vi "Main.vi"(11 "Module Admin":refnum<class "Delacor_lib_QMH_Module Admin.lvclass">) -> ()   [LabVIEW 2018, in "MainInterface.lvlib"]
doc: "This template is based off of the Queued Message Handler design pattern and the Queued Message Handler project template that ships with LabVIEW.\n\nThe main difference is that the queue is private to this module and communication between modules is performed via Broadcast and Request events.\n\nRequest events are wrapped in public API methods and are handled in the Event Handling Loop (EHL) of this VI. Any module can register for Broadcast events sent by this module. The EHL generates messages based on user interface actions.\n\nThe Message Handling Loop (MHL) processes messages generated by the EHL, or by other messages. The messages are string values, so new messages can be added easily to the Message Cases case structure in the MHL. Each message cluster can also provide an optional value for Message Data, which is a variant that can be converted to whatever message-specific data is required.\n_____\nBased on DQMH Project Template 7.0.1.1316."
uses:
  MainInterface.lvlib
  <vilib>/Delacor/Delacor QMH/Libraries/Module Admin_class/Delacor_lib_QMH_Module Admin.lvclass
  User Interface/Status Light Bar.ctl
  User Interface/User Interface.lvclass
  <vilib>/Delacor/Delacor QMH/Libraries/Message Queue_class/Delacor_lib_QMH_Message Queue.lvclass/Delacor_lib_QMH_Message Queue.ctl
  Launch Function Argument.ctl
  Stop Argument--cluster.ctl
  Register Window Argument--cluster.ctl
  <vilib>/Delacor/Delacor QMH/Libraries/Message Queue_class/Delacor_lib_QMH_Message Queue.lvclass
  Unregister Window Argument--cluster.ctl
  Is Window Opened Argument--cluster.ctl
  Is Window Opened (Reply Payload)--cluster.ctl
  Disbale Item Argument--cluster.ctl
  Enable Item Argument--cluster.ctl
  <vilib>/Utility/miscctls.llb/LVPointTypeDef.ctl
  <vilib>/Delacor/Delacor QMH/Libraries/Module Admin_class/Delacor_lib_QMH_Module Admin.lvclass/Delacor_lib_QMH_Module Admin.ctl
  <vilib>/Delacor/Delacor QMH/Libraries/Message Queue_class/Delacor_lib_QMH_Enqueue Message (Single).vi
  <vilib>/Delacor/Delacor QMH/Libraries/Module Admin_class/Delacor_lib_QMH_Get External Launch.vi
  ModuleInterface/ModuleInterface.lvlib
panel:
  in  "Status Light Bar":T1=enum."Green"
  in  "min":bool
  in  "close":bool
  out "error out":errorcluster
  out "Status":string
  in  "Simulate MHL Error":bool
  in  "Simulate EHL Error":bool
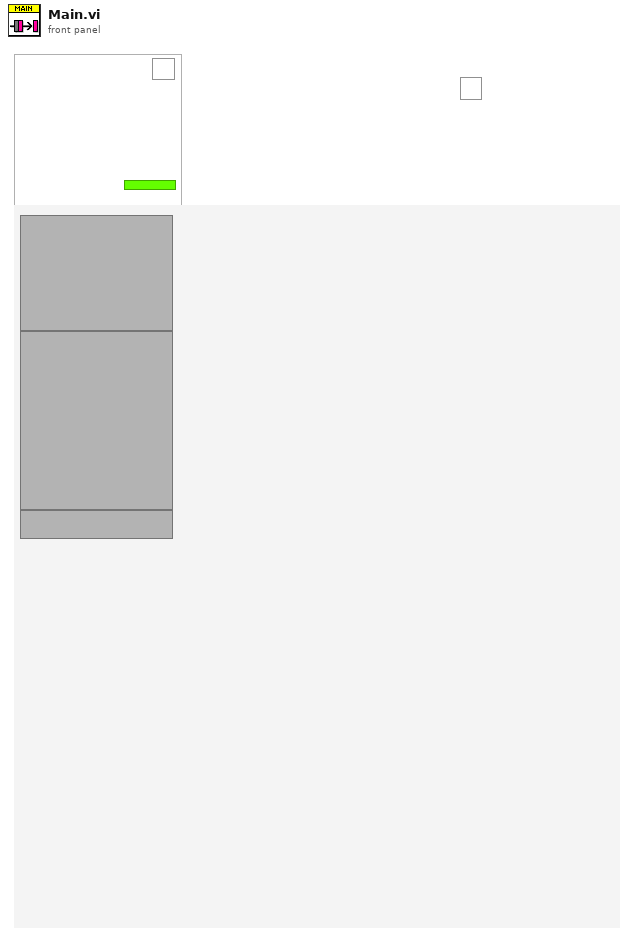
[diagram p1: front panel]
types:
  T1 = typedef "MainInterface.lvlib/User Interface.lvclass/Status Light Bar.ctl" = enum32{"Red", "Yellow", "Green"}
  T2 = typedef "MainInterface.lvlib/Request Events--cluster.ctl" = cluster{"Stop Module":refnum<user-event>, "Show Panel":refnum<user-event>, "Hide Panel":refnum<user-event>, "Get Module Execution Status":refnum<user-event>, "Show Diagram":refnum<user-event>, "Register Window":refnum<user-event>, "Unregister Window":refnum<user-event>, "Is Window Opened":refnum<user-event>, "Disbale Item":refnum<user-event>, "Enable Item":refnum<user-event>}
  T3 = typedef "ModuleInterface.lvlib/ModuleDefinition.ctl" = cluster{"模块名称":string, "项定义":T4[]}
  T4 = typedef "ModuleInterface.lvlib/FunctionItem.ctl" = cluster{"项名":string, "符号图形路径":path}
  T5 = typedef "ModuleInterface.lvlib/Broadcast Events--cluster.ctl" = cluster{"Module Did Init":refnum<user-event>, "Status Updated":refnum<user-event>, "Error Reported":refnum<user-event>, "Module Did Stop":refnum<user-event>, "Update Module Execution Status":refnum<user-event>, "Function Selected":refnum<user-event>, "Window Size Changed":refnum<user-event>}
  T6 = typedef "MainInterface.lvlib/Launch Function Argument.ctl" = cluster{"Module ID":i32, "Module Name":string, "Item Name":string}
  T7 = enum32{"invalid lock state", "Not Locked", "Locked (No Password)", "Password-protected"}
  T8 = typedef "MainInterface.lvlib/Stop Argument--cluster.ctl" = cluster{"Origin":string, "Exit via Stop Module Req?":bool, "Wait for Module to stop?":bool}
  T9 = typedef "MainInterface.lvlib/Register Window Argument--cluster.ctl" = cluster{"Name":string, "Reference":refnum<vi>, "Message Queue":refnum<class "Delacor_lib_QMH_Message Queue.lvclass">}
  T10 = typedef "MainInterface.lvlib/Unregister Window Argument--cluster.ctl" = cluster{"Window Name":string}
  T11 = typedef "MainInterface.lvlib/Is Window Opened Argument--cluster.ctl" = cluster{"Window Name":string, "Wait Notifier":refnum<notifier>, "wait for reply":bool}
  T12 = typedef "MainInterface.lvlib/Disbale Item Argument--cluster.ctl" = cluster{"Module Name":string, "Item Name":string}
  T13 = typedef "MainInterface.lvlib/Enable Item Argument--cluster.ctl" = cluster{"Module Name":string, "Item Name":string}
  T14 = enum32{"Invalid", "Standard", "Closed", "Hidden", "Minimized", "Maximized"}
  T15 = typedef "MainInterface.lvlib/Is Window Opened (Reply Payload)--cluster.ctl" = cluster{"Opened？":bool, "error":errorcluster}
  T16 = typedef "LVPointTypeDef.ctl" = cluster{"Horizontal":i16, "Vertical":i16}
  T17 = typedef "LVRectTypeDef.ctl" = cluster{"Left":i16, "Top":i16, "Right":i16, "Bottom":i16}
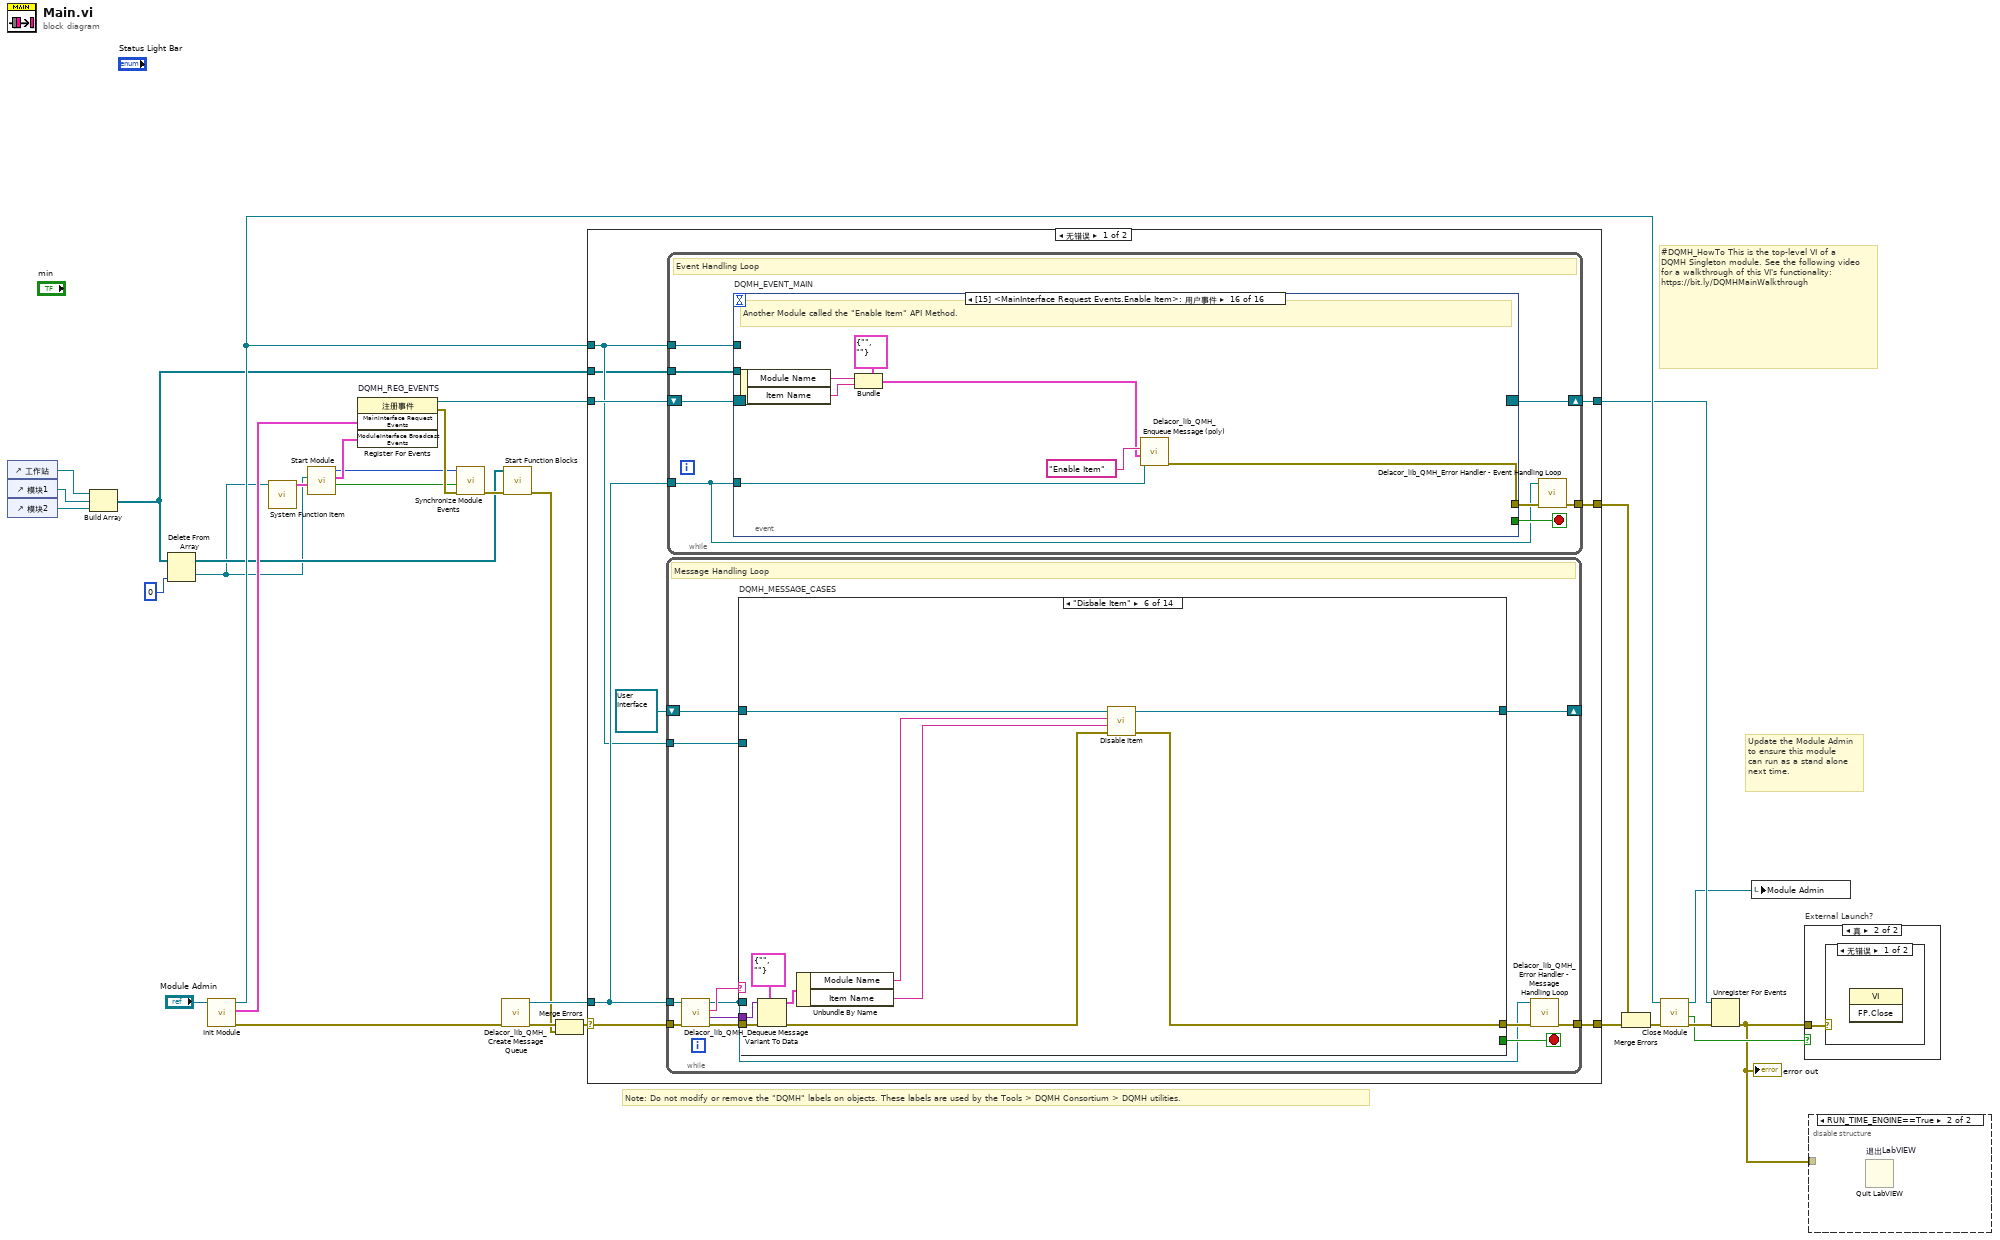
[diagram p0: block diagram]
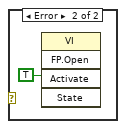
[diagram p4: hidden frame]
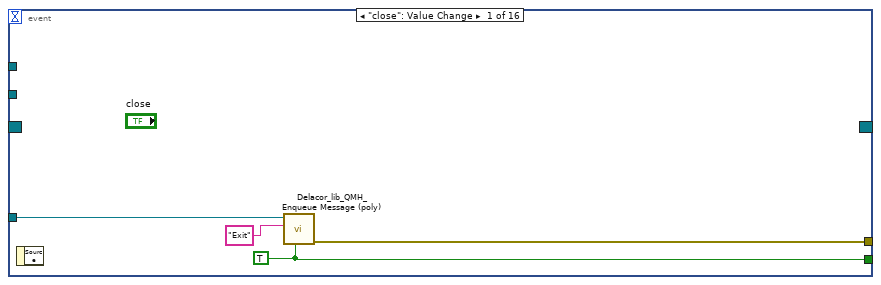
[diagram p5: hidden frame]
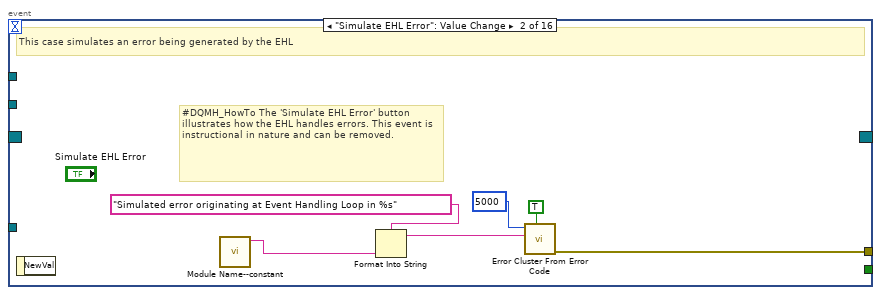
[diagram p6: hidden frame]
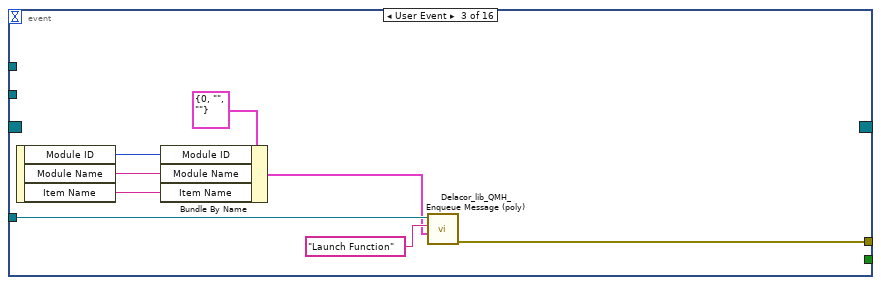
[diagram p7: hidden frame]
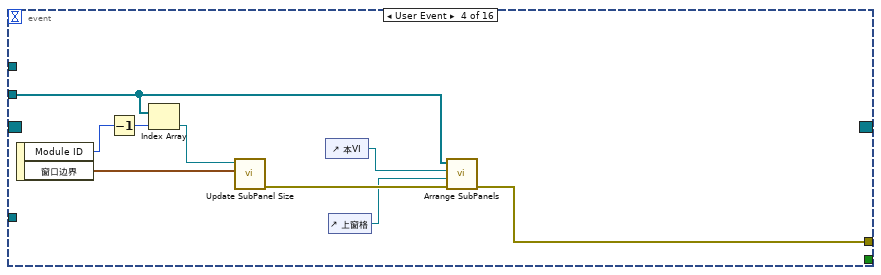
[diagram p8: hidden frame]
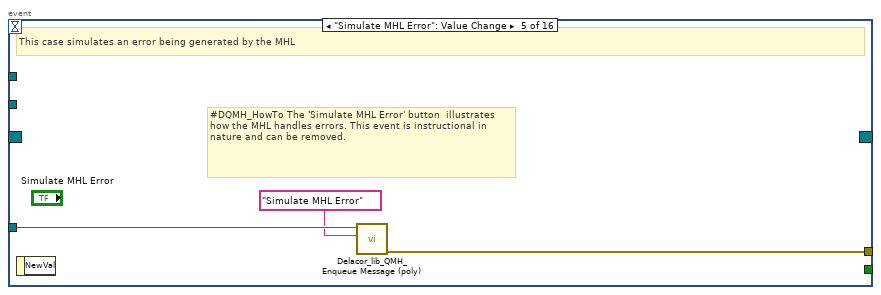
[diagram p9: hidden frame]
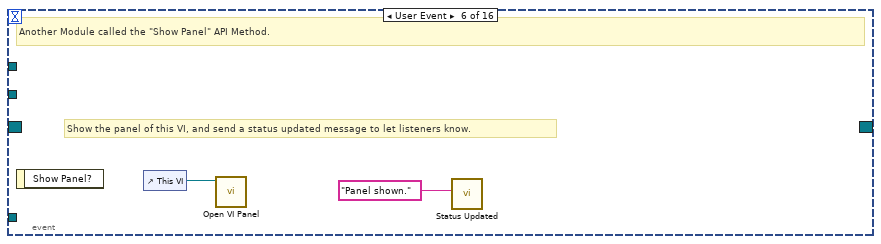
[diagram p10: hidden frame]
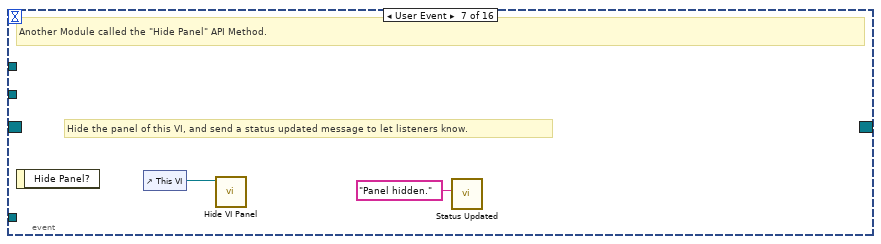
[diagram p11: hidden frame]
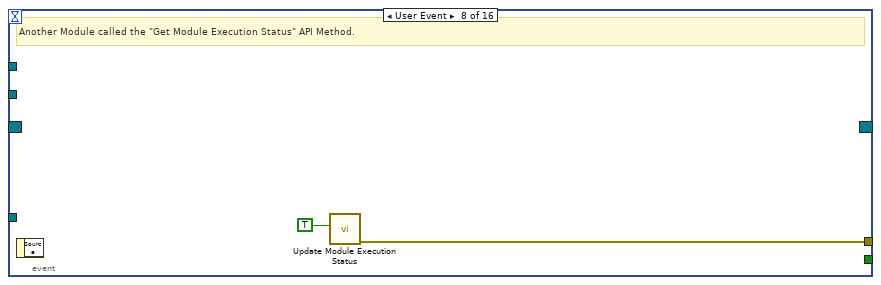
[diagram p12: hidden frame]
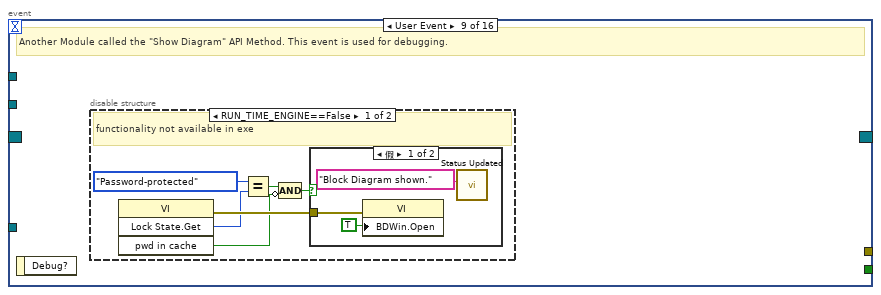
[diagram p13: hidden frame]
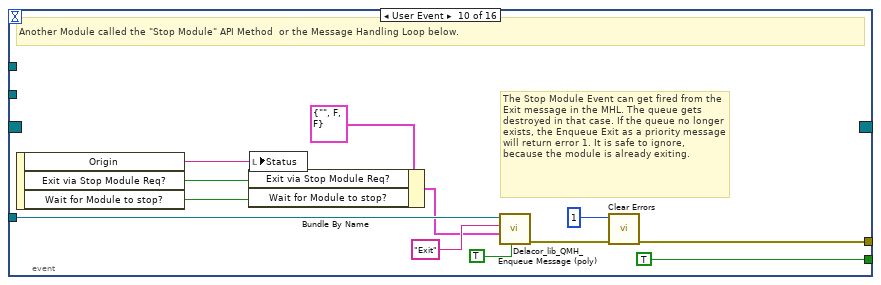
[diagram p16: hidden frame]
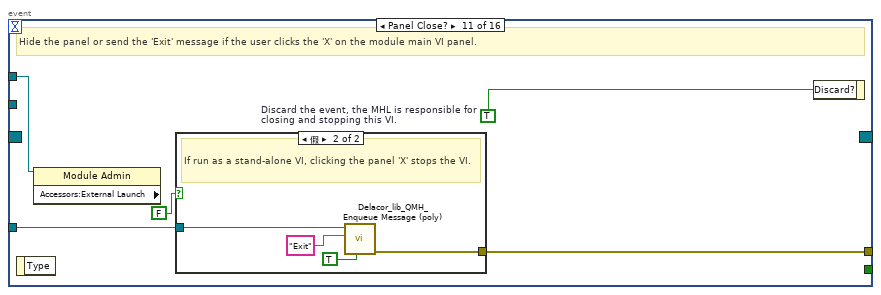
[diagram p17: hidden frame]
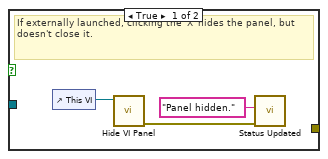
[diagram p18: hidden frame]
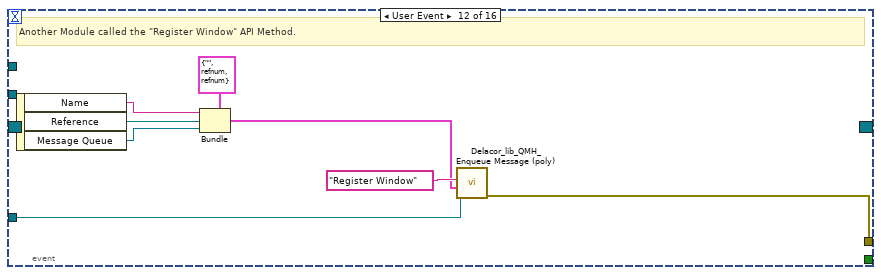
[diagram p19: hidden frame]
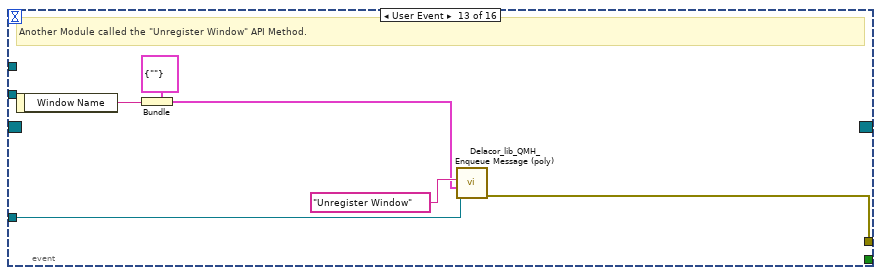
[diagram p20: hidden frame]
diagram:
  # "#DQMH_HowTo This is the top-level VI of a DQMH Singleton module. See the following video for a walkthrough of this VI's functionality: https://bit.ly/DQMHMainWalkthrough"
  # "Note: Do not modify or remove the \"DQMH\" labels on objects. These labels are used by the Tools > DQMH Consortium > DQMH utilities."
  # "Update the Module Admin to ensure this module can run as a stand alone next time."
  n1 = control-ref of="工作站"() -> (w9:refnum<vi>)
  n2 = control-ref of="模块1"() -> (w8:refnum<vi>)
  n3 = control-ref of="模块2"() -> (w6:refnum<vi>)
  n4 = Build Array(w9, w8, w6) -> (w7:refnum<vi>[])
  n5 = Delete From Array(array=w7, index=0 ("索引")) -> (deleted portion=w1:refnum<vi>, array with subset deleted=w4:refnum<vi>[])  [unwired: 1 in]
  n6 = call "Init Module.vi"("Singleton Module Admin in"="Module Admin") -> ("error out"=w29:errorcluster, "MainInterface Request Events"=w20:T2, "Singleton Module Admin out"=w23:refnum<class "Delacor_lib_QMH_Module Admin.lvclass">)  [unwired: 8 in]
  n7 = call "System Function Item.vi"("rSubPane"=w1) -> ("模块定义"=w16:T3)  [unwired: 10 in]
  n8 = call "Start Module.vi"("模块定义"=w16, "rSubPanel"=w1) -> ("Wait for Event Sync?"=w13:bool, "ModuleInterface Broadcast Events"=w15:T5, "Module ID"=w12:i32)  [unwired: 6 in, 1 out]
  n9 = register-events "DQMH_REG_EVENTS"(w20, w15) -> (reference out=w21:refnum<event-registration>, error out=w14:errorcluster)  [unwired: 2 in]
  n10 = call "Synchronize Module Events.vi"("error in"=w14, "Wait for Event Sync?"=w13, "Module ID in"=w12) -> ("error out"=w11:errorcluster)  [unwired: 7 in, 1 out]
  n11 = call <vilib>:"Delacor_lib_QMH_Create Message Queue.vi"("error in"=w29) -> ("error out"=w25:errorcluster, "Message Queue"=w19:refnum<class "Delacor_lib_QMH_Message Queue.lvclass">)  [unwired: 9 in]
  n12 = call "Start Function Blocks.vi"("错误输入（无错误）"=w11, "子面板数组"=w4) -> ("错误输出"=w10:errorcluster)  [unwired: 9 in]
  n13 = Merge Errors(w25, w10) -> (w24:errorcluster)
  n14 = case shown="无错误" w24 {
    selector: w24 -> [w37 w325]
    tunnel: [w39 w324] -> w30
    tunnel: [w36 w323] -> w22
    tunnel: w21 -> [w35 w323]
    tunnel: w19 -> [w34 w318]
    tunnel: [w38 _] -> w27
    tunnel: w23 -> [w33 w319]
    tunnel: w7 -> [w32 _]
    frame No Error {
      n15 = while {
        tunnel: w34 -> [w153]
        shift-right: [w161] -> _
        shift-left: refnum<class "User Interface.lvclass"> refnum ("MainInterface.lvlib:User Interface.lvclass") -> [w162]
        tunnel: w37 -> [w164]
        tunnel: [w156] -> w39
        tunnel: w33 -> [w157]
        stop <- w160 stop-if-true
        # "Message Handling Loop"
        n16 = call-dynamic "Delacor_lib_QMH_Dequeue Message.vi"("error in"=w164, "Message Queue in"=w153) -> ("error out"=w163:errorcluster, "Message Data"=w158:variant, "Message"=w159:string, "Message Queue out"=w154:refnum<class "Delacor_lib_QMH_Message Queue.lvclass">)  [unwired: 6 in]
        n17 = case "DQMH_MESSAGE_CASES" shown="\"Disbale Item\"" w159 {
          selector: w159 -> [_ _ _ _ _ _ _ _ _ _ _ _ _ w313]
          tunnel: w154 -> [_ _ _ _ _ _ _ _ _ _ _ w276 w301 _]
          tunnel: w163 -> [w167 w191 w199 w208 w222 w234 w244 w247 w256 w263 w272 w283 w307 w316]
          tunnel: [w186 w191 w192 w200 w209 w225 w235 w246 w255 w263 w271 w279 w302 w317] -> w155
          tunnel: w162 -> [w177 w190 w196 w204 w214 w233 w240 w245 w249 w262 w269 w278 w293 w314]
          tunnel: [w169 w190 w195 w203 w213 w229 w239 w245 w248 w262 w269 w278 w292 w314] -> w161
          tunnel: [_ _ _ _ _ _ _ _ _ _ _ _ w300 _] -> w160
          tunnel: w158 -> [_ _ w198 w207 w221 w232 w243 _ w254 _ _ w277 w299 _]
          tunnel: w157 -> [w178 _ _ _ _ _ _ _ _ _ _ w275 w294 _]
          frame "Initialize" {
            w170 = T16 {"Horizontal"=0, "Vertical"=0} ("原点")
            w168 = "Initial Message" ("Initial Message")
            # "背景色RGB为，244，244，244"
            # "Initialize - Any operation that needs to be done before the module can receive messages. Synchronize Caller Events.vi will inform Start Module.vi that the module has launched and is ready to receive messages. Module Did Init.vi will broadcast that the module initialized."
            n18 = call "Synchronize Caller Events.vi"("error in"=w167, "Singleton Module Admin in"=w178) -> ("error out"=w187:errorcluster, "Singleton Module Admin out"=w174:refnum<class "Delacor_lib_QMH_Module Admin.lvclass">)  [unwired: 8 in]
            n19 = property on="Property Node" class="Module Admin"(reference=w174) -> ("Accessors:External Launch"=w182:bool)  [unwired: 1 in, 2 out]
            n20 = Select(t=T14."Hidden" ("State"), s=w182, f=T14."Standard" ("State")) -> (s? t:f=w179:T14)
            n21 = call "Module Name--constant.vi"() -> ("Module Name"=w185:string)  [unwired: 11 in]
            n22 = property on="Property Node" class="VI"("Front Panel.Title"=w185) -> (reference out=w184:refnum<vi>, error out=w189:errorcluster)  [unwired: 2 in]
            n23 = invoke on="Invoke Node" class="VI" method="FP.Open"(reference=w184, error in=w189, "State"=w179) -> (reference out=w183:refnum<vi>, error out=w188:errorcluster)  [unwired: 2 in, 3 out]
            n24 = call "Initialize.vi"("error in (no error)"=w167, "Status"=w168, "User Interface 输入"=w177) -> ("error out"=w165:errorcluster, "User Interface 输出"=w169:refnum<class "User Interface.lvclass">)  [unwired: 7 in]
            n25 = invoke on="Invoke Node" class="VI" method="FP.Center"(reference=w183, error in=w188) -> ()  [unwired: 1 in, 3 out]
            n26 = Merge Errors(w165, w187) -> (w166:errorcluster)
            n27 = control-ref of="下窗格"() -> (w173:refnum<vi>)
            n28 = control-ref of="上窗格"() -> (w172:refnum<vi>)
            n29 = property class="Pane"(reference=w173, "PaneColor"=u32 16053492 ("窗格颜色"), "Origin"=w170) -> ()  [unwired: 1 in, 2 out]
            n30 = property class="Pane"(reference=w172, "Origin"=w170) -> ()  [unwired: 1 in, 2 out]
            n31 = call "FramelessFP Drop-In.vi"("Pane in"=w172) -> ()  [unwired: 10 in, 1 out]
            n32 = call "Module Name--constant.vi"() -> ("Module Name"=w175:string)  [unwired: 11 in]
            n33 = call "Module Did Init.vi"("error in"=w166, "Initialized?"=TRUE, "Origin"=w175) -> ("error out"=w186:errorcluster)  [unwired: 8 in]
            "Status" <- w168
          }
          frame "---Module Specific---" {
            # "Separator -- The following cases handle messages specific to this Module."
          }
          frame "Register Window" {
            # "登记已打开的窗口的信息"
            n34 = Variant To Data(error in=w199, type=T9 {"Name"="", "Reference"=refnum, "Message Queue"=refnum} ("Register Window Argument"), Variant=w198) -> (data=w194:T9, error out=w193:errorcluster)
            n35 = call "Register Window.vi"("error in (no error)"=w193, "New Window"=w194, "User Interface 输入"=w196) -> ("error out"=w192:errorcluster, "User Interface 输出"=w195:refnum<class "User Interface.lvclass">)  [unwired: 7 in]
          }
          frame "Unregister Window" {
            # "从登记信息中清除相应的窗口信息"
            n36 = Variant To Data(error in=w208, type=T10 {"Window Name"=""} ("Unregister Window Argument"), Variant=w207) -> (data=w205:T10, error out=w201:errorcluster)
            n37 = Unbundle By Name(w205) -> ("Window Name"=w202:string)
            n38 = call "Unregister Window.vi"("error in (no error)"=w201, "Window Name"=w202, "User Interface 输入"=w204) -> ("error out"=w200:errorcluster, "User Interface 输出"=w203:refnum<class "User Interface.lvclass">)  [unwired: 7 in]
          }
          frame "Is Window Opened" {
            # "检查窗口是否已打开？"
            n39 = Variant To Data(error in=w222, type=T11 {"Window Name"="", "Wait Notifier"=refnum, "wait for reply"=FALSE} ("Is Window Opened Argument"), Variant=w221) -> (data=w219:T11, error out=w210:errorcluster)
            n40 = Unbundle By Name(w219) -> ("Window Name"=w212:string, "Wait Notifier"=w218:refnum<notifier>, "wait for reply"=w217:bool)
            n41 = call "Check Window Existence.vi"("error in (no error)"=w210, "Window Name"=w212, "User Interface 输入"=w214) -> ("error out"=w209:errorcluster, "已存在？"=w211:bool, "User Interface 输出"=w213:refnum<class "User Interface.lvclass">)  [unwired: 6 in]
            n42 = Bundle By Name(cluster=T15 {"Opened？"=FALSE, "error"={"status"=FALSE, "code"=0, "source"=""}} ("Is Window Opened (Reply Payload)"), "Opened？"=w211) -> (w216:T15)
            n43 = case "DQMH_FIRE_NOTIFIER" shown="真" w217 {
              tunnel: w218 -> [_ w224]
              tunnel: w216 -> [_ w223]
              frame False {
              }
              frame True {
                n44 = Send Notification(notification=w223, notifier=w224) -> ()  [unwired: 1 in, 2 out]
              }
            }
          }
          frame "Disbale Item" {
            n45 = Variant To Data(error in=w234, type=T12 {"Module Name"="", "Item Name"=""} ("Disbale Item Argument"), Variant=w232) -> (data=w230:T12, error out=w226:errorcluster)
            n46 = Unbundle By Name(w230) -> ("Module Name"=w228:string, "Item Name"=w227:string)
            n47 = call "Disable Item.vi"("error in (no error)"=w226, "Item Name"=w227, "Module Name"=w228, "User Interface 输入"=w233) -> ("error out"=w225:errorcluster, "User Interface 输出"=w229:refnum<class "User Interface.lvclass">)  [unwired: 6 in]
          }
          frame "Enable Item" {
            n48 = Variant To Data(error in=w244, type=T13 {"Module Name"="", "Item Name"=""} ("Enable Item Argument"), Variant=w243) -> (data=w241:T13, error out=w236:errorcluster)
            n49 = Unbundle By Name(w241) -> ("Module Name"=w238:string, "Item Name"=w237:string)
            n50 = call "Enable Item.vi"("error in (no error)"=w236, "Item Name"=w237, "Module Name"=w238, "User Interface 输入"=w240) -> ("error out"=w235:errorcluster, "User Interface 输出"=w239:refnum<class "User Interface.lvclass">)  [unwired: 6 in]
          }
          frame "---Copy This Frame---" {
            # "Duplicate this frame when creating new messages.  Change this comment in the duplicated frame to describe this message."
            n51 = Merge Errors(w247) -> (w246:errorcluster)
          }
          frame "Launch Function" {
            # "Duplicate this frame when creating new messages.  Change this comment in the duplicated frame to describe this message."
            n52 = Variant To Data(type=T6 {"Module ID"=0, "Module Name"="", "Item Name"=""} ("Launch Function Argument"), Variant=w254) -> (data=w252:T6)  [unwired: 1 in, 1 out]
            n53 = Unbundle By Name(w252) -> ("Item Name"=w250:string, "Module Name"=w251:string)
            n54 = case shown="\"退出\"" w250 {
              selector: w250 -> [w260 _]
              tunnel: w251 -> [w259 _]
              tunnel: w249 -> [w257 w261]
              tunnel: [w257 w261] -> w248
              frame "假", Default {
                n55 = call "Generate Window Name.vi"("Module Name"=w259, "Item Name"=w260) -> ("Window Name"=w258:string)  [unwired: 9 in]
                n56 = One Button Dialog(message=w258) -> ()  [unwired: 1 in, 1 out]
              }
              frame "退出" {
                n57 = call "Stop Module.vi"() -> ()  [unwired: 11 in, 1 out]
              }
            }
            n58 = Merge Errors(w256) -> (w255:errorcluster)
          }
          frame "---Exit and Error Handling---" {
            # "Separator - The following cases handle errors and exit messages."
          }
          frame "Simulate MHL Error" {
            # "#DQMH_HowTo The 'Simulate MHL Error' button  illustrates how the MHL handles errors. This event is instructional in nature and can be removed."
            # "Simulate an error occurring at the MHL"
            n59 = call "Module Name--constant.vi"() -> ("Module Name"=w265:string)  [unwired: 11 in]
            n60 = Format Into String(format string="Simulated error originating at Message Handling Loop in %s", w265) -> (resulting string=w266:string)  [unwired: 2 in, 1 out]
            n61 = call <vilib>:"Error Cluster From Error Code.vi"("show call chain? (False)"=TRUE, "error message (\"\")"=w266, "error code (0)"=5001) -> ("error out"=w270:errorcluster)  [unwired: 6 in]
            n62 = Merge Errors(w272, w270) -> (w271:errorcluster)
          }
          frame "Error" {
            # "#CodeRecommended - If the module is running in standalone mode (External Launch = FALSE), this code will pop up an error dialog and call the 'Exit' message if an error occurs. Add more fine-grained error management here."
            # "Error - Check the error message data and respond accordingly. This message is sent by the \"Error Handler\" VIs at the end of each loop in this application."
            n63 = property on="Property Node" class="Module Admin"(reference=w275) -> ("Accessors:External Launch"=w274:bool)  [unwired: 1 in, 2 out]
            n64 = Variant To Data(error in=w283, type=errorcluster {"status"=FALSE, "code"=0, "source"=""} ("error constant"), Variant=w277) -> (data=w273:errorcluster, error out=w281:errorcluster)
            n65 = local write "error out"(w273) -> ()
            n66 = call "Error Reported.vi"("Error"=w273) -> ()  [unwired: 10 in, 1 out]
            n67 = case shown="假" w274 {
              tunnel: [w288 _] -> w280
              tunnel: w276 -> [w286 _]
              tunnel: w273 -> [w287 _]
              frame False {
                n68 = disable-structure shown="Default" {
                  disable-tunnel: w287 -> [w289 _]
                  frame condition #0 (active) {
                    # "If the module is running standalone, then pop up an error dialog and call the \"Exit\" message."
                    n69 = call <vilib>:"Simple Error Handler.vi"("error in (no error)"=w289) -> ()  [unwired: 4 in, 5 out]
                  }
                  frame condition #1 {
                    # "To prevent the Simple Error Handler VI from being loaded (e.g. when deploying to a Real-Time target), add the Conditional Disable Symbol \"DQMH_Disable_SEH\" to your project and set it to TRUE."
                  }
                }
                n70 = call-poly <vilib>:"Delacor_lib_QMH_Enqueue Message (poly).vi"("Priority Message? (F)"=TRUE, "Message"="Exit", "Message Queue in"=w286) -> ("error out"=w288:errorcluster)  [unwired: 7 in, 1 out]
              }
              frame True {
                # "If the module was launched externally, calling the Error Reported broadcast VI is the only action performed by the \"Error\" message. The module's caller can then process the error appropriately."
              }
            }
            n71 = Merge Errors(w281, w280) -> (w279:errorcluster)
          }
          frame "Exit" {
            w298 = 91  # 91: not all Exit messages will have an argument
            w300 = TRUE  # Stop the VI
            # "Release the message queue reference"
            # "Exit - Exit the application."
            n72 = Variant To Data(error in=w307, type=T8 {"Origin"="", "Exit via Stop Module Req?"=FALSE, "Wait for Module to stop?"=FALSE} ("Stop Argument"), Variant=w299) -> (data=w296:T8, error out=w304:errorcluster)
            n73 = call <vilib>:"Clear Errors.vi"("error in (no error)"=w304, "specific error code to clear (0: all)"=w298) -> ("error out"=w306:errorcluster)  [unwired: 4 in, 1 out]
            n74 = control-ref of="This VI"() -> (w295:refnum<vi>)
            n75 = call-dynamic "Delacor_lib_QMH_Release Message Queue.vi"("error in"=w306, "Message Queue"=w301) -> ("error out"=w305:errorcluster)  [unwired: 9 in]
            n76 = call "Handle Exit.vi"("Stop Argument"=w296, "Admin in"=w294, "VI reference"=w295) -> ("error out"=w303:errorcluster)  [unwired: 7 in, 1 out]
            n77 = call "Force Close Window.vi"("User Interface 输入"=w293) -> ("error out"=w291:errorcluster, "User Interface 输出"=w292:refnum<class "User Interface.lvclass">)  [unwired: 9 in]
            n78 = Merge Errors(w291, w305, w303) -> (w302:errorcluster)
            n79 = call "Stop Module.vi"("Module ID"=-1) -> ()  [unwired: 10 in, 1 out]
            n80 = call "Error Reported.vi"("Error"=w302) -> ()  [unwired: 10 in, 1 out]
          }
          frame Default {
            # "'Default' case only runs if there is a message that isn't defined in any of the other cases.  Output a programming error."
            n81 = call "Module Name--constant.vi"() -> ("Module Name"=w312:string)  [unwired: 11 in]
            n82 = Format Into String(format string="The invalid message string \"%s\" was received in the Message Handling Loop for module \"%s\".", w313, w312) -> (resulting string=w308:string)  [unwired: 2 in, 1 out]
            n83 = call <vilib>:"Error Cluster From Error Code.vi"("show call chain? (False)"=TRUE, "error message (\"\")"=w308, "error code (0)"=1) -> ("error out"=w315:errorcluster)  [unwired: 6 in]
            n84 = Merge Errors(w316, w315) -> (w317:errorcluster)
          }
        }
        n85 = call-dynamic "Delacor_lib_QMH_Error Handler - Message Handling Loop.vi"("error in"=w155, "Message Queue in"=w154) -> ("dup error in"=w156:errorcluster)  [unwired: 8 in, 1 out]
      }
      n86 = while {
        tunnel: w34 -> [w41]
        shift-right: [w44] -> w36
        shift-left: w35 -> [w45]
        tunnel: [w46] -> w38
        tunnel: w33 -> [w42]
        tunnel: w32 -> [w40]
        stop <- w43 stop-if-true
        # "Event Handling Loop"
        n87 = event "DQMH_EVENT_MAIN" shown="[15] <MainInterface Request Events.Enable Item>: 用户事件" {
          selector: w45 -> [_ _ _ _ _ _ _ _ _ _ _ _ _ _ _ _]
          dyn-events: [_ _ _ _ _ _ _ _ _ _ _ _ _ _ _ _] -> w44
          timeout: _ -> [_ _ _ _ _ _ _ _ _ _ _ _ _ _ _ _]
          tunnel: [w49 _ _ _ _ _ _ _ _ TRUE ("Discard?") _ _ _ _ _ _] -> w43
          tunnel: w41 -> [w50 _ w61 _ w76 _ _ _ _ w100 w107 w124 w130 w138 w145 w152]
          tunnel: [w48 w57 w58 w66 w77 _ _ w83 _ w103 w109 w120 w125 w131 w139 w146] -> w47
          tunnel: w42 -> [_ _ _ _ _ _ _ _ _ _ w106 _ _ _ _ _]
          tunnel: w40 -> [_ _ _ w70 _ _ _ _ _ _ _ _ _ _ _ _]
          event "close": Value Change {
            w49 = TRUE
            n88 = event-data() -> ()  [unwired: 1 in, 1 out]
            n89 = call-poly <vilib>:"Delacor_lib_QMH_Enqueue Message (poly).vi"("Priority Message? (F)"=w49, "Message"="Exit", "Message Queue in"=w50) -> ("error out"=w48:errorcluster)  [unwired: 7 in, 1 out]
          }
          event "Simulate EHL Error": Value Change {
            # "#DQMH_HowTo The 'Simulate EHL Error' button  illustrates how the EHL handles errors. This event is instructional in nature and can be removed."
            # "This case simulates an error being generated by the EHL"
            n90 = event-data() -> ()  [unwired: 1 in, 1 out]
            n91 = call "Module Name--constant.vi"() -> ("Module Name"=w54:string)  [unwired: 11 in]
            n92 = Format Into String(format string="Simulated error originating at Event Handling Loop in %s", w54) -> (resulting string=w55:string)  [unwired: 2 in, 1 out]
            n93 = call <vilib>:"Error Cluster From Error Code.vi"("show call chain? (False)"=TRUE, "error message (\"\")"=w55, "error code (0)"=5000) -> ("error out"=w57:errorcluster)  [unwired: 6 in]
          }
          event User Event {
            n94 = event-data() -> ("Module ID"=w64:i32, "Module Name"=w63:string, "Item Name"=w62:string)  [unwired: 1 in]
            n95 = Bundle By Name(cluster=T6 {"Module ID"=0, "Module Name"="", "Item Name"=""} ("Launch Function Argument"), "Module ID"=w64, "Module Name"=w63, "Item Name"=w62) -> (w59:T6)
            n96 = call-poly <vilib>:"Delacor_lib_QMH_Enqueue Message (poly).vi"("Message Data"=w59, "Message"="Launch Function", "Message Queue in"=w61) -> ("error out"=w58:errorcluster)  [unwired: 7 in, 1 out]
          }
          event User Event {
            n97 = event-data() -> ("Module ID"=w74:i32, "窗口边界"=w72:T17)  [unwired: 1 in]
            n98 = Decrement(x=w74) -> (x-1=w71:i32)
            n99 = Index Array(array=w70, index=w71) -> (element=w73:refnum<vi>)
            n100 = call "Update SubPanel Size.vi"("窗口边界"=w72, "SubPanel输入"=w73) -> ("错误输出"=w69:errorcluster)  [unwired: 9 in]
            n101 = control-ref of="本VI"() -> (w68:refnum<vi>)
            n102 = control-ref of="上窗格"() -> (w67:refnum<vi>)
            n103 = call "Arrange SubPanels.vi"("错误输入（无错误）"=w69, "上窗格"=w67, "VI引用句柄"=w68, "rSubPanes"=w70) -> ("错误输出"=w66:errorcluster)  [unwired: 7 in]
          }
          event "Simulate MHL Error": Value Change {
            # "#DQMH_HowTo The 'Simulate MHL Error' button  illustrates how the MHL handles errors. This event is instructional in nature and can be removed."
            # "This case simulates an error being generated by the MHL"
            n104 = event-data() -> ()  [unwired: 1 in, 1 out]
            n105 = call-poly <vilib>:"Delacor_lib_QMH_Enqueue Message (poly).vi"("Message"="Simulate MHL Error", "Message Queue in"=w76) -> ("error out"=w77:errorcluster)  [unwired: 8 in, 1 out]
          }
          event User Event {
            # "Show the panel of this VI, and send a status updated message to let listeners know."
            # "Another Module called the \"Show Panel\" API Method."
            n106 = event-data() -> ()  [unwired: 1 in, 1 out]
            n107 = control-ref of="This VI"() -> (w79:refnum<vi>)
            n108 = call "Open VI Panel.vi"("VI"=w79) -> ()  [unwired: 10 in, 1 out]
            n109 = call "Status Updated.vi"("Status"="Panel shown." ("format string")) -> ()  [unwired: 10 in, 1 out]
          }
          event User Event {
            # "Hide the panel of this VI, and send a status updated message to let listeners know."
            # "Another Module called the \"Hide Panel\" API Method."
            n110 = event-data() -> ()  [unwired: 1 in, 1 out]
            n111 = control-ref of="This VI"() -> (w81:refnum<vi>)
            n112 = call "Hide VI Panel.vi"("VI"=w81) -> ()  [unwired: 10 in, 1 out]
            n113 = call "Status Updated.vi"("Status"="Panel hidden." ("format string")) -> ()  [unwired: 10 in, 1 out]
          }
          event User Event {
            # "Another Module called the \"Get Module Execution Status\" API Method."
            n114 = event-data() -> ()  [unwired: 1 in, 1 out]
            n115 = call "Update Module Execution Status.vi"("Running?"=TRUE) -> ("error out"=w83:errorcluster)  [unwired: 10 in]
          }
          event User Event {
            # "Another Module called the \"Show Diagram\" API Method. This event is used for debugging."
            n116 = event-data() -> ()  [unwired: 1 in, 1 out]
            n117 = disable-structure shown="RUN_TIME_ENGINE==False" {
              frame condition #0 (active) {
                # "functionality not available in exe"
                n118 = invoke on="Invoke Node" class="VI" method="Lock State.Get"() -> (error out=w89:errorcluster, "Get Lock State"=w88:T7, "pwd in cache"=w85:bool)  [unwired: 4 in, 1 out]
                n119 = Equal?(x=T7."Password-protected", y=w88) -> (x = y?=w86:bool)
                n120 = Compound Arithmetic op=AND(w86, invert w85) -> (w84:bool)
                n121 = case shown="假" w84 {
                  tunnel: w89 -> [w92 _]
                  frame False {
                    n122 = property on="Property Node" class="VI"(error in=w92, "BDWin.Open"=TRUE ("Block Diagram Window:Open")) -> ()  [unwired: 1 in, 2 out]
                    n123 = call "Status Updated.vi"("Status"="Block Diagram shown." ("format string")) -> ()  [unwired: 10 in, 1 out]
                  }
                  frame True {
                    # "Password-protected VI, and the password is not in the cache. Do not show the diagram."
                  }
                }
              }
              frame condition #1 {
              }
            }
          }
          event User Event {
            # "The Stop Module Event can get fired from the Exit message in the MHL. The queue gets destroyed in that case. If the queue no longer exists, the Enqueue Exit as a priority message will return error 1. It is safe to ignore, because the module is already exiting."
            # "Another Module called the \"Stop Module\" API Method  or the Message Handling Loop below."
            n124 = event-data() -> ("Origin"=w99:string, "Exit via Stop Module Req?"=w95:bool, "Wait for Module to stop?"=w94:bool)  [unwired: 1 in]
            n125 = Bundle By Name(cluster=T8 {"Origin"="", "Exit via Stop Module Req?"=FALSE, "Wait for Module to stop?"=FALSE} ("Stop Argument"), "Exit via Stop Module Req?"=w95, "Wait for Module to stop?"=w94) -> (w93:T8)
            n126 = local write "Status"(w99) -> ()
            n127 = call-poly <vilib>:"Delacor_lib_QMH_Enqueue Message (poly).vi"("Priority Message? (F)"=TRUE, "Message Data"=w93, "Message"="Exit", "Message Queue in"=w100) -> ("error out"=w104:errorcluster)  [unwired: 6 in, 1 out]
            n128 = call <vilib>:"Clear Errors.vi"("error in (no error)"=w104, "specific error code to clear (0: all)"=1) -> ("error out"=w103:errorcluster)  [unwired: 4 in, 1 out]
          }
          event Panel Close? {
            w108 = TRUE  # Discard the event, the MHL is responsible for closing and stopping this VI.
            # "Hide the panel or send the 'Exit' message if the user clicks the 'X' on the module main VI panel."
            n129 = event-data() -> ()  [unwired: 1 in, 1 out]
            n130 = property on="Property Node" class="Module Admin" props=["Accessors:External Launch"](reference=w106) -> ()  [unwired: 1 in, 3 out]
            n131 = case shown="假" FALSE {
              tunnel: w107 -> [_ w115]
              tunnel: [_ w116] -> w109
              frame True {
                # "If externally launched, clicking the 'X' hides the panel, but doesn't close it."
                n132 = control-ref of="This VI"() -> (w112:refnum<vi>)
                n133 = call "Hide VI Panel.vi"("VI"=w112) -> ("error out"=w110:errorcluster)  [unwired: 10 in]
                n134 = call "Status Updated.vi"("error in"=w110, "Status"="Panel hidden." ("format string")) -> ()  [unwired: 9 in, 1 out]
              }
              frame False {
                # "If run as a stand-alone VI, clicking the panel 'X' stops the VI."
                n135 = call-poly <vilib>:"Delacor_lib_QMH_Enqueue Message (poly).vi"("Priority Message? (F)"=TRUE, "Message"="Exit", "Message Queue in"=w115) -> ("error out"=w116:errorcluster)  [unwired: 7 in, 1 out]
              }
            }
            n136 = event-data ("Event Filter Node")("Discard?"=w108) -> ()  [unwired: 1 in, 1 out]
          }
          event User Event {
            # "Another Module called the \"Register Window\" API Method."
            n137 = event-data() -> ("Name"=w119:string, "Reference"=w118:refnum<vi>, "Message Queue"=w117:refnum<class "Delacor_lib_QMH_Message Queue.lvclass">)  [unwired: 1 in]
            n138 = Bundle(cluster=T9 {"Name"="", "Reference"=refnum, "Message Queue"=refnum} ("Register Window Argument"), "Name"=w119, "Reference"=w118, "Message Queue"=w117) -> (w121:T9)
            n139 = call-poly <vilib>:"Delacor_lib_QMH_Enqueue Message (poly).vi"("Message Data"=w121, "Message"="Register Window", "Message Queue in"=w124) -> ("error out"=w120:errorcluster)  [unwired: 7 in, 1 out]
          }
          event User Event {
            # "Another Module called the \"Unregister Window\" API Method."
            n140 = event-data() -> ("Window Name"=w126:string)  [unwired: 1 in]
            n141 = Bundle(cluster=T10 {"Window Name"=""} ("Unregister Window Argument"), "Window Name"=w126) -> (w127:T10)
            n142 = call-poly <vilib>:"Delacor_lib_QMH_Enqueue Message (poly).vi"("Message Data"=w127, "Message"="Unregister Window", "Message Queue in"=w130) -> ("error out"=w125:errorcluster)  [unwired: 7 in, 1 out]
          }
          event User Event {
            # "Another Module called the \"Is Window Opened\" API Method."
            n143 = event-data() -> ("Window Name"=w134:string, "Wait Notifier"=w133:refnum<notifier>, "wait for reply"=w132:bool)  [unwired: 1 in]
            n144 = Bundle(cluster=T11 {"Window Name"="", "Wait Notifier"=refnum, "wait for reply"=FALSE} ("Is Window Opened Argument"), "Window Name"=w134, "Wait Notifier"=w133, "wait for reply"=w132) -> (w135:T11)
            n145 = call-poly <vilib>:"Delacor_lib_QMH_Enqueue Message (poly).vi"("Message Data"=w135, "Message"="Is Window Opened", "Message Queue in"=w138) -> ("error out"=w131:errorcluster)  [unwired: 7 in, 1 out]
          }
          event User Event {
            # "Another Module called the \"Disbale Item\" API Method."
            n146 = event-data() -> ("Module Name"=w141:string, "Item Name"=w140:string)  [unwired: 1 in]
            n147 = Bundle(cluster=T12 {"Module Name"="", "Item Name"=""} ("Disbale Item Argument"), "Module Name"=w141, "Item Name"=w140) -> (w142:T12)
            n148 = call-poly <vilib>:"Delacor_lib_QMH_Enqueue Message (poly).vi"("Message Data"=w142, "Message"="Disbale Item", "Message Queue in"=w145) -> ("error out"=w139:errorcluster)  [unwired: 7 in, 1 out]
          }
          event User Event {
            # "Another Module called the \"Enable Item\" API Method."
            n149 = event-data() -> ("Module Name"=w148:string, "Item Name"=w147:string)  [unwired: 1 in]
            n150 = Bundle(cluster=T13 {"Module Name"="", "Item Name"=""} ("Enable Item Argument"), "Module Name"=w148, "Item Name"=w147) -> (w149:T13)
            n151 = call-poly <vilib>:"Delacor_lib_QMH_Enqueue Message (poly).vi"("Message Data"=w149, "Message"="Enable Item", "Message Queue in"=w152) -> ("error out"=w146:errorcluster)  [unwired: 7 in, 1 out]
          }
        }
        n152 = call-dynamic "Delacor_lib_QMH_Error Handler - Event Handling Loop.vi"("error in"=w47, "Message Queue in"=w41) -> ("dup error in"=w46:errorcluster)  [unwired: 8 in, 1 out]
      }
    }
    frame Error {
      # "Synchronize Caller Events.vi will inform Start Module.vi that the module has launched and will let the code calling Start Module.vi register for broadcasts and would permit the caller receive the broadcast that an error occurred at launch time."
      n153 = call-dynamic "Delacor_lib_QMH_Release Message Queue.vi"("error in"=w325, "Message Queue"=w318) -> ("error out"=w324:errorcluster)  [unwired: 9 in]
      n154 = call "Synchronize Caller Events.vi"("Singleton Module Admin in"=w319) -> ("error out"=w326:errorcluster)  [unwired: 9 in, 1 out]
      n155 = call "Module Name--constant.vi"() -> ("Module Name"=w322:string)  [unwired: 11 in]
      n156 = Format Into String(format string="An error occurred during initialization. %s is no longer running.", w322) -> (resulting string=w320:string)  [unwired: 2 in, 1 out]
      n157 = Merge Errors(w324, w326) -> (w327:errorcluster)
      n158 = call "Error Reported.vi"("Additional Information"=w320, "Error"=w327) -> ()  [unwired: 9 in, 1 out]
    }
  }
  n159 = Merge Errors(w27, w30) -> (w26:errorcluster)
  n160 = call "Close Module.vi"("error in"=w26, "Module Admin in"=w23) -> ("error out"=w28:errorcluster, "External Launch"=w3:bool, "Module Admin out"=w17:refnum<class "Delacor_lib_QMH_Module Admin.lvclass">)  [unwired: 7 in]
  n161 = Unregister For Events(event registration refnum=w22, error in=w28) -> (error out=w2:errorcluster)
  "error out" <- w2
  n162 = local write "Module Admin"(w17) -> ()
  n163 = case "External Launch?" shown="真" w3 {
    tunnel: w2 -> [_ w328]
    frame False {
    }
    frame True {
      n164 = case shown="无错误" w328 {
        frame No Error {
          n165 = invoke class="VI" method="FP.Close"() -> ()  [unwired: 3 in, 3 out]
        }
        frame Error {
          n166 = invoke class="VI" method="FP.Open"("Activate"=TRUE ("Activate?")) -> ()  [unwired: 4 in, 5 out]
        }
      }
    }
  }
  n167 = disable-structure shown="RUN_TIME_ENGINE==True" {
    disable-tunnel: w2 -> [_ _]
    frame condition #0 (active) {
    }
    frame condition #1 {
      n168 = Quit LabVIEW "退出LabVIEW"() -> ()  [unwired: 1 in]
    }
  }
